vi "T7MOD_Read_FLOAT32_Register.vi"(8 "error in":errorcluster, 9 "LabJack FLOAT32 Register":i32=55124, 10 "Remote Port":u16=502, 11 "Remote IP Address":string="192.168.1.15") -> (0 "error out":errorcluster, 1 "Read At":timestamp, 2 "Raw Data Read":u16[](array[numeric]), 3 "Read FLOAT32":sgl)   [LabVIEW 2018]
panel:
  # "Output"
  # "TCP Parameters"
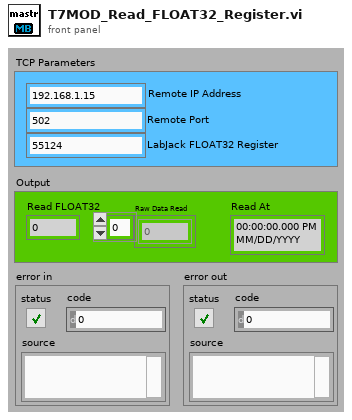
[diagram p1: front panel]
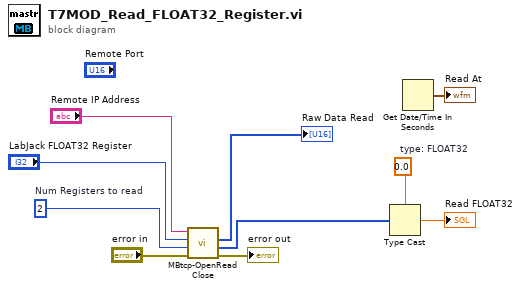
[diagram p0: block diagram]
diagram:
  w10 = sgl 0.0  # type: FLOAT32
  w5 = 2  # Num Registers to read
  n1 = call "MBtcp-OpenReadClose.vi"("error in (no error)"="error in", "nRegisters"=w5, "RegisterAddr"="LabJack FLOAT32 Register", "IP Address(:port)"="Remote IP Address") -> ("error out"=→"error out":errorcluster, "32bitValues"=w2:u32[], "16bitValues"=→"Raw Data Read":u16[])  [unwired: 5 in]
  n2 = Type Cast(type=w10, x=w2) -> (*(type *) &x=→"Read FLOAT32":sgl)
  n3 = Get Date/Time In Seconds() -> (seconds since 1Jan1904=→"Read At":timestamp)
